vi "Write Val.vi"(8 "error in (no error)":errorcluster, 10 "Val":bool, 11 "Update Switch MSG in":refnum<class "Update Switch MSG.lvclass">) -> (0 "error out":errorcluster, 3 "Update Switch MSG out":refnum<class "Update Switch MSG.lvclass">)   [LabVIEW 2014, in "Update Switch MSG.lvclass"]
uses:
  Update Switch MSG.lvclass
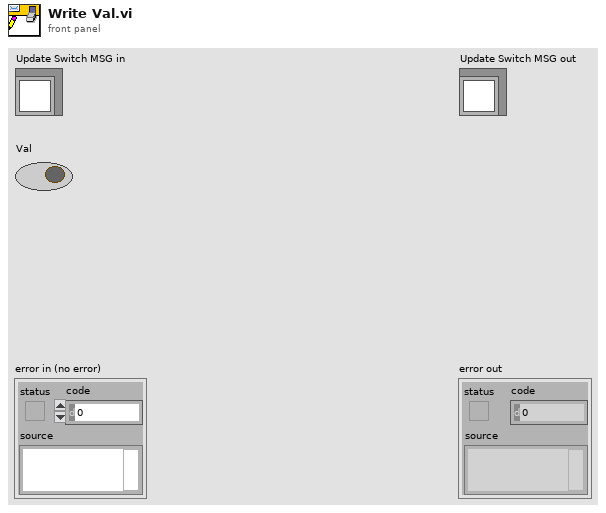
[diagram p1: front panel]
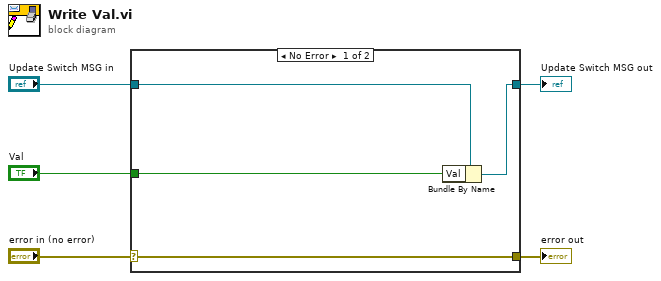
[diagram p0: block diagram]
diagram:
  n1 = case shown="No Error" "error in (no error)" {
    selector: "error in (no error)" -> [w9 w10]
    tunnel: [w9 w10] -> w4
    tunnel: [w7 w11] -> w2
    tunnel: "Update Switch MSG in" -> [w8 w11]
    tunnel: "Val" -> [w6 _]
    frame No Error {
      n2 = Bundle By Name(cluster=w8, "Val"=w6) -> (w7:refnum<class "Update Switch MSG.lvclass">)
    }
    frame Error {
    }
  }
  "error out" <- w4
  "Update Switch MSG out" <- w2
